vi "Get Ref.vi"(8 "error in (no error)":errorcluster, 11 "BetterMultiListboxHandle in":refnum<class "BetterMultiListboxHandle.lvclass">) -> (0 "error out":errorcluster, 2 "Tree/LB/MCL ref":refnum<vi>, 3 "BetterMultiListboxHandle out":refnum<class "BetterMultiListboxHandle.lvclass">)   [LabVIEW 2020, in "BetterDragAndDrop.lvlib" / "BetterMultiListboxHandle.lvclass"]
uses:
  BetterMultiListboxHandle.lvclass
  BetterMultiListboxHandle.lvclass/BetterMultiListboxHandle.ctl
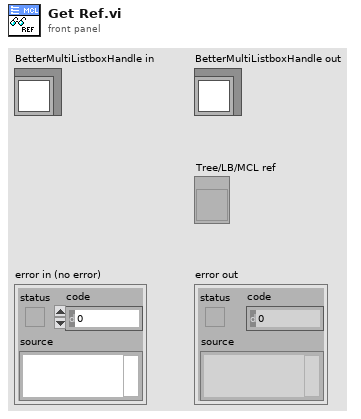
[diagram p1: front panel]
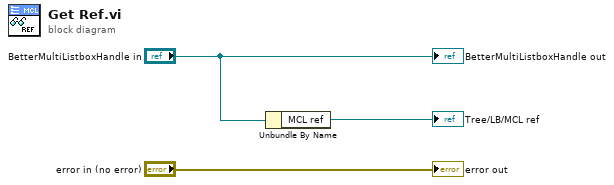
[diagram p0: block diagram]
diagram:
  n1 = Unbundle By Name("BetterMultiListboxHandle in") -> ("MCL ref"=→"Tree/LB/MCL ref":refnum<vi>)
  "error out" <- "error in (no error)"
  "BetterMultiListboxHandle out" <- "BetterMultiListboxHandle in"
